vi "Open Handle.vi"(6 "verify server(true)":bool=TRUE, 7 "cookie file":path, 8 "error in (no error)":errorcluster, 9 "password":string, 10 "username":string, 11 "HTTP Client Base in":refnum<class "LabVIEW HTTP Client.lvclass">) -> (0 "error out":errorcluster, 3 "HTTP Client Base out":refnum<class "LabVIEW HTTP Client.lvclass">)   [LabVIEW 2021, in "HTTP Client Abstract.lvlib" / "LabVIEW HTTP Client.lvclass"]
uses:
  LabVIEW HTTP Client.lvclass
  LabVIEW HTTP Client.lvclass/LabVIEW HTTP Client.ctl
  <vilib>/httpClient/LabVIEWHTTPClient.lvlib
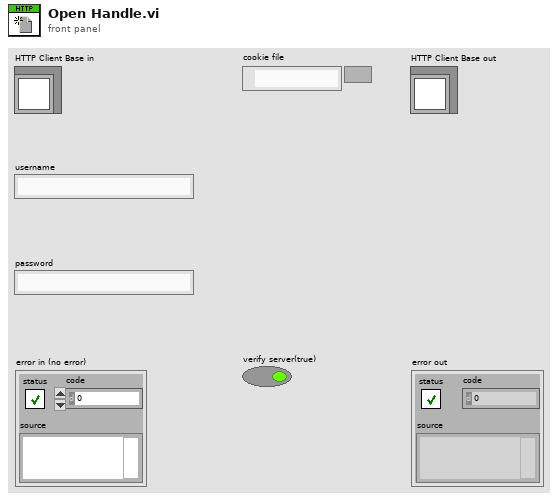
[diagram p1: front panel]
types:
  T1 = typedef "LabVIEWHTTPClient.lvlib/ClientHandle.ctl" = refnum<k1>
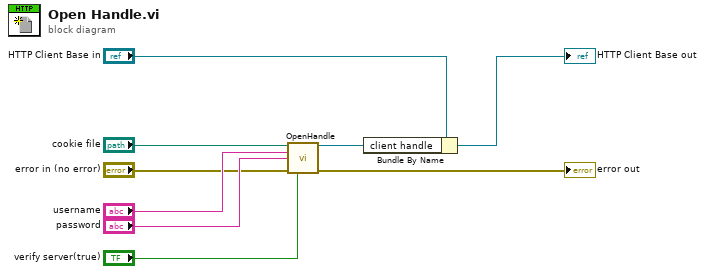
[diagram p0: block diagram]
diagram:
  n1 = call <vilib>:"OpenHandle.vi"("cookie file"="cookie file", "username"="username", "password"="password", "error in (no error)"="error in (no error)", "verify server(true)"="verify server(true)") -> ("client handle out"=w2:T1, "error out"=→"error out":errorcluster)  [unwired: 9 in]
  n2 = Bundle By Name(cluster="HTTP Client Base in", "client handle"=w2) -> (→"HTTP Client Base out":refnum<class "LabVIEW HTTP Client.lvclass">)
